vi "Teleop.vi"(10 "Match Info":T1={"Autonomous Elapsed Seconds"=0.0, "TeleOp Elapsed Seconds"=0.0, "Disabled Elapsed Seconds"=0.0, "Visited Autonomous"=FALSE, "Visited TeleOp"=FALSE, "Visited Disabled"=FALSE, "Autonomous Settings"={"Autonomous Style"=enum."Independent", "VI Refnum"=refnum}}, 11 "Call Context":T2) -> ()   [LabVIEW 2016]
doc: "This VI is called for each TeleOp packet received from the DS where the robot is not disabled. It is often used to read from the joysticks and update I/O or to update setpoints for timed control loops. It should complete and return within 20 milliseconds or it may miss DS packets."
uses:
  <vilib>/Rock Robotics/WPI/DriverStation/WPI_DriverStationDerivedRobotMode.ctl
  <vilib>/Rock Robotics/WPI/DriverStation/WPI_DriverStationMatch Info.ctl
  Refname/Controllers.ctl
  Refname/Refname to String (Controllers).vi
  <vilib>/Rock Robotics/WPI/Utilities/WPI_GetSetVariantRefNum.vi
  Robot Global Data.vi
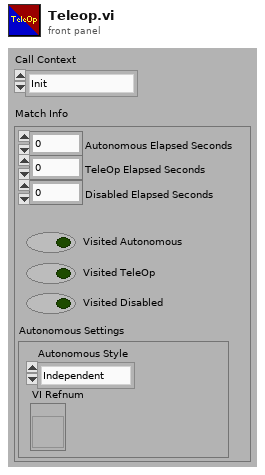
[diagram p1: front panel]
types:
  T1 = typedef "WPI_DriverStationMatch Info.ctl" = cluster{"Autonomous Elapsed Seconds":dbl, "TeleOp Elapsed Seconds":dbl, "Disabled Elapsed Seconds":dbl, "Visited Autonomous":bool, "Visited TeleOp":bool, "Visited Disabled":bool, "Autonomous Settings":cluster{"Autonomous Style":enum16{"Iterative", "Independent"}, "VI Refnum":refnum<vi>}}
  T2 = typedef "WPI_DriverStationDerivedRobotMode.ctl" = enum16{"Init", "Execute", "Stop"}
  T3 = cluster{"X":dbl, "Y":dbl, "Z":dbl, "Straight Drive":bool, "Reverse Drive":bool, "Low Sensitivity":bool, "X Button":bool, "Button B":bool}
  T4 = typedef "Controllers.ctl" = enum16{"Controller 0", "Controller 1", "Controller 2"}
  T5 = typedef "WPI_JoystickDevRef.ctl" = cluster{"Device":T6}
  T6 = typedef "WPI_JoystickDeviceEnum.ctl" = enum16{"USB 0", "USB 1", "USB 2", "USB 3", "USB 4", "USB 5"}
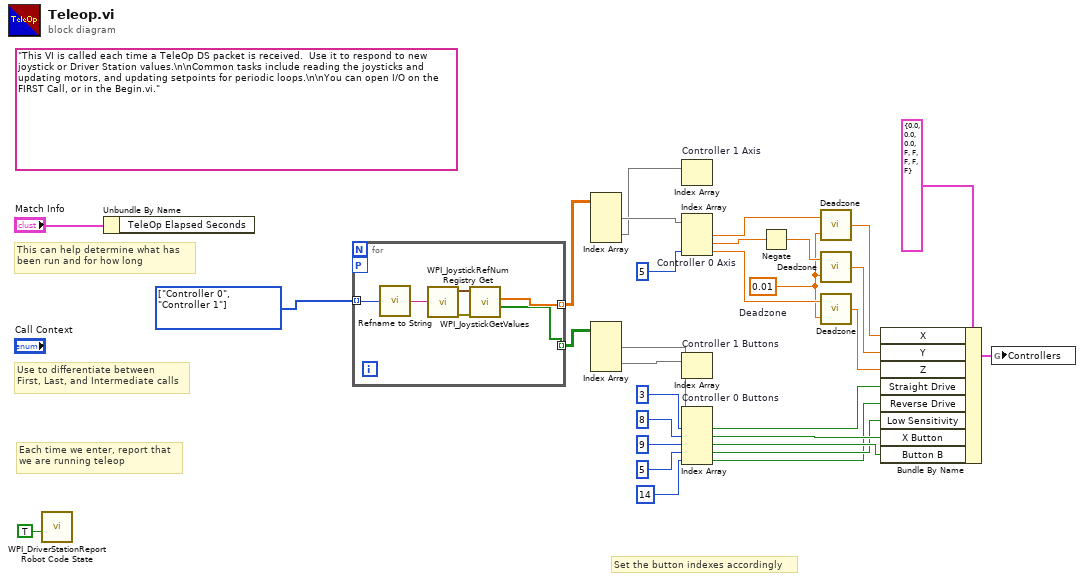
[diagram p0: block diagram]
diagram:
  w1 = T3 {"X"=0.0, "Y"=0.0, "Z"=0.0, "Straight Drive"=FALSE, "Reverse Drive"=FALSE, "Low Sensitivity"=FALSE, "X Button"=FALSE, "Button B"=FALSE} ("Controllers")
  w2 = 0.01  # Deadzone
  w27 = T4[] [enum."Controller 0", enum."Controller 1"] items=["Controller 0", "Controller 1", "Controller 2"]
  (unwired) "This VI is called each time a TeleOp DS packet is received.  Use it to respond to new joystick or Driver Station values.\n\nCommon tasks include reading the joysticks and updating motors, and updating setpoints for periodic loops.\n\nYou can open I/O on the FIRST Call, or in the Begin.vi."
  # "Set the button indexes accordingly"
  # "Each time we enter, report that\nwe are running teleop"
  # "Use to differentiate between\nFirst, Last, and Intermediate calls"
  # "This can help determine what has\nbeen run and for how long"
  n1 = call <vilib>:"WPI_DriverStationReport Robot Code State.vi"("TeleOp"=TRUE ("Autonomous")) -> ()  [unwired: 10 in, 1 out]
  n2 = Unbundle By Name("Match Info") -> ()  [unwired: 1 out]
  n3 = for {
    workers-P: _ -> [_]
    tunnel: w27 -> [w35] mode=indexing
    tunnel: [w31] -> w26 mode=indexing
    tunnel: [w30] -> w21 mode=indexing
    n4 = call-poly "Refname to String.vi"("Enum"=w35) -> ("resulting string"=w32:string)
    n5 = call <vilib>:"WPI_JoystickRefNum Registry Get.vi"("refnum name"=w32) -> ("error out"=w33:errorcluster, "JoystickDevRef"=w34:T5)  [unwired: 9 in]
    n6 = call <vilib>:"WPI_JoystickGetValues.vi"("error in (no error)"=w33, "JoystickDevRef"=w34) -> ("Buttons"=w30:bool[], "Axes"=w31:dbl[])  [unwired: 5 in, 3 out]
  }
  n7 = Index Array(array=w26) -> (element #1=w25:dbl[], element #2=w24:dbl[])  [unwired: 4 in]
  n8 = Index Array(array=w21) -> (element #1=w20:bool[], element #2=w19:bool[])  [unwired: 4 in]
  n9 = Index Array "Controller 1 Axis"(array=w24) -> ()  [unwired: 1 in, 1 out]
  n10 = Index Array "Controller 0 Axis"(array=w25, index #3=5 ("index")) -> (element #1=w7:dbl, element #2=w22:dbl, element #3=w4:dbl)  [unwired: 2 in]
  n11 = Index Array "Controller 1 Buttons"(array=w19) -> ()  [unwired: 1 in, 1 out]
  n12 = Index Array "Controller 0 Buttons"(array=w20, index #1=3 ("index"), index #2=8 ("index"), index #3=9 ("index"), index #4=5 ("index"), index #5=14 ("index")) -> (element #1=w13:bool, element #2=w12:bool, element #3=w11:bool, element #4=w10:bool, element #5=w9:bool)
  n13 = Negate(x=w22) -> (-x=w6:dbl)
  n14 = call "Deadzone.vi"("Deadzone"=w2, "Value"=w7) -> ("Numeric"=w8:dbl)
  n15 = call "Deadzone.vi"("Deadzone"=w2, "Value"=w6) -> ("Numeric"=w5:dbl)
  n16 = call "Deadzone.vi"("Deadzone"=w2, "Value"=w4) -> ("Numeric"=w3:dbl)
  n17 = Bundle By Name(cluster=w1, "X"=w8, "Y"=w5, "Z"=w3, "Straight Drive"=w13, "Reverse Drive"=w9, "Low Sensitivity"=w10, "X Button"=w12, "Button B"=w11) -> ()  [unwired: 1 out]
  n18 = global write "Robot Global Data.vi" "Controllers"(w1) -> ()
